vi "RFID Get ID.vi"(11 "ComPort":refnum<visa-resource-name>="COM10") -> (0 "error out":errorcluster, 3 "received":string)   [LabVIEW 2018]
uses:
  <vilib>/Instr/_visa.llb/VISA Configure Serial Port (Instr).vi
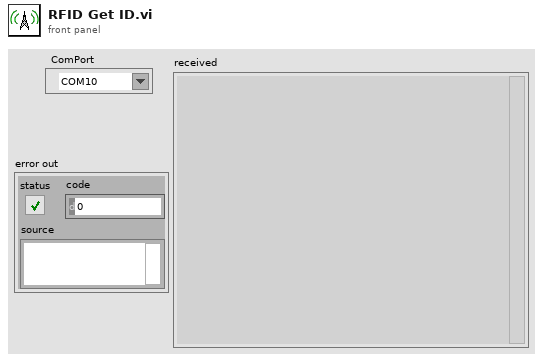
[diagram p1: front panel]
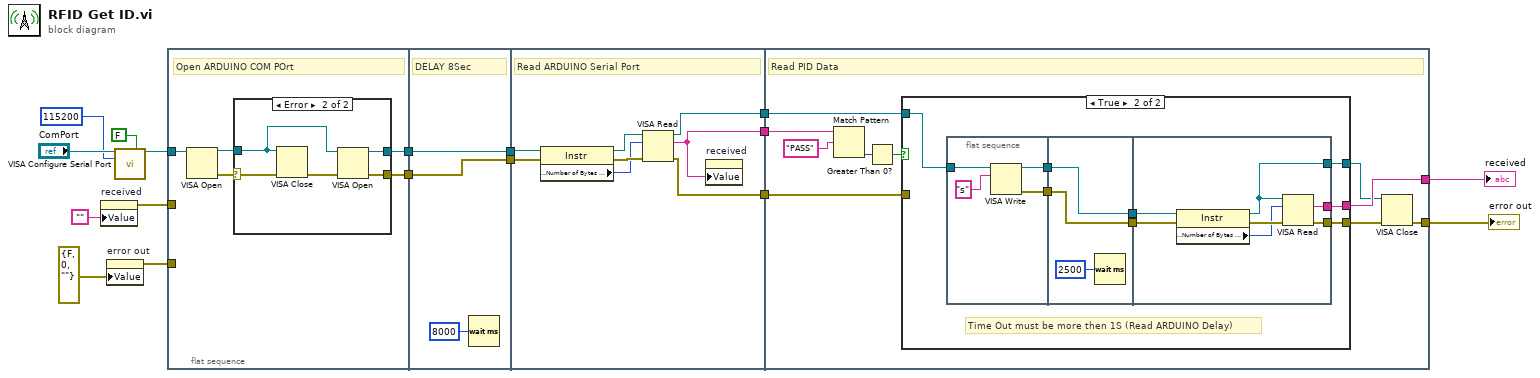
[diagram p0: block diagram]
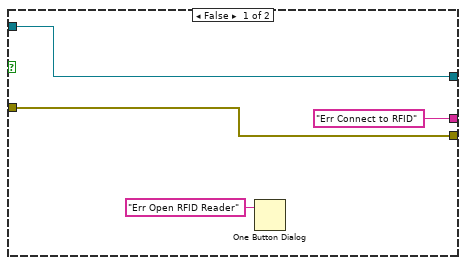
[diagram p3: hidden frame]
diagram:
  n1 = property on="received" class="Str"("Value"="") -> (error out=w16:errorcluster)  [unwired: 2 in, 1 out]
  n2 = property on="error out" class="Clust (strict)"("Value"=errorcluster {"status"=FALSE, "code"=0, "source"=""} ("error out")) -> (error out=w15:errorcluster)  [unwired: 2 in, 1 out]
  n3 = call-poly "VISA Configure Serial Port"("VISA resource name"="ComPort", "Enable Termination\nChar (T)"=FALSE ("Enable Termination\nChar (T)"), "baud rate (9600)"=u32 115200 ("Serial Settings:Baud Rate")) -> ("VISA resource name out"=w4:refnum<visa-resource-name>)  [unwired: 11 in, 1 out]
  n4 = flat-sequence {
    tunnel: w4 -> [w20]
    tunnel: w16 -> [_]
    tunnel: w15 -> [_]
    tunnel: [w19] -> w12
    tunnel: [w18] -> w10
    tunnel: [w31] -> w13
    tunnel: w12 -> [w31]
    tunnel: [w30] -> w11
    tunnel: w10 -> [w30]
    tunnel: w13 -> [w37]
    tunnel: w11 -> [w36]
    tunnel: [w35] -> w9
    tunnel: [w34] -> w8
    tunnel: [w33] -> w6
    tunnel: w9 -> [w50]
    tunnel: w8 -> [w46]
    tunnel: [w45] -> w7
    tunnel: [w43] -> w1
    tunnel: w6 -> [w44]
    frame #0 {
      # "Open ARDUINO COM POrt"
      n5 = VISA Open(VISA resource name=w20) -> (VISA resource name=w22:refnum<visa-resource-name>, error out=w21:errorcluster)  [unwired: 4 in]
      n6 = case shown="Error" w21 {
        selector: w21 -> [w23 w29]
        tunnel: w22 -> [w24 w27]
        tunnel: [w24 w26] -> w19
        tunnel: [w23 w25] -> w18
        frame No Error {
        }
        frame Error {
          n7 = VISA Close(VISA resource name=w27, error in (no error)=w29) -> (error out=w28:errorcluster)
          n8 = VISA Open(error in (no error)=w28, VISA resource name=w27) -> (VISA resource name=w26:refnum<visa-resource-name>, error out=w25:errorcluster)  [unwired: 3 in]
        }
      }
    }
    frame #1 {
      # "DELAY 8Sec"
      n9 = Wait (ms)(milliseconds to wait=u32 8000) -> ()  [unwired: 1 out]
    }
    frame #2 {
      # "Read ARDUINO Serial Port"
      n10 = property class="Instr"(reference=w37, error in=w36) -> (reference out=w39:refnum<visa-resource-name>, error out=w40:errorcluster, "Serial Settings:Number of Bytes at Serial Port"=w38:u32)
      n11 = VISA Read(VISA resource name=w39, byte count=w38, error in (no error)=w40) -> (VISA resource name out=w34:refnum<visa-resource-name>, read buffer=w35:string, error out=w33:errorcluster)  [unwired: 1 out]
      n12 = property on="received" class="Str"("Value"=w35) -> ()  [unwired: 2 in, 2 out]
    }
    frame #3 {
      # "Read PID Data"
      n13 = Match Pattern(string=w50, regular expression="PASS") -> (offset past match=w48:i32)  [unwired: 1 in, 3 out]
      n14 = Greater Than 0?(x=w48) -> (x > 0?=w47:bool)
      n15 = case shown="True" w47 {
        tunnel: w46 -> [w51 w58]
        tunnel: ["Err Connect to RFID" ("read buffer") w57] -> w45
        tunnel: [w53 w56] -> w42
        tunnel: w44 -> [w53 _]
        tunnel: [w51 w55] -> w41
        frame False {
          n16 = One Button Dialog(message="Err Open RFID Reader") -> ()  [unwired: 1 in, 1 out]
        }
        frame True {
          # "Time Out must be more then 1S (Read ARDUINO Delay)"
          n17 = flat-sequence {
            tunnel: w58 -> [w66]
            tunnel: [w64] -> w62
            tunnel: [w63] -> w61
            tunnel: w62 -> [w68]
            tunnel: w61 -> [w67]
            tunnel: [w68] -> w60
            tunnel: [w67] -> w59
            tunnel: w60 -> [w74]
            tunnel: w59 -> [w73]
            tunnel: [w72] -> w56
            tunnel: [w71] -> w57
            tunnel: [w70] -> w55
            frame #0 {
              n18 = VISA Write(VISA resource name=w66, write buffer="s") -> (VISA resource name out=w64:refnum<visa-resource-name>, error out=w63:errorcluster)  [unwired: 1 in, 1 out]
            }
            frame #1 {
              n19 = Wait (ms)(milliseconds to wait=u32 2500) -> ()  [unwired: 1 out]
            }
            frame #2 {
              n20 = property class="Instr"(reference=w74, error in=w73) -> (reference out=w70:refnum<visa-resource-name>, error out=w76:errorcluster, "Serial Settings:Number of Bytes at Serial Port"=w75:u32)
              n21 = VISA Read(VISA resource name=w70, byte count=w75, error in (no error)=w76) -> (read buffer=w71:string, error out=w72:errorcluster)  [unwired: 2 out]
            }
          }
        }
      }
      n22 = VISA Close(VISA resource name=w41, error in (no error)=w42) -> (error out=w43:errorcluster)
    }
  }
  "received" <- w7
  "error out" <- w1
